vi "Actor Core.vi"(8 "error in":errorcluster, 11 "Nested in":refnum<class "UI_Up_Down.lvclass">) -> (0 "error out":errorcluster, 3 "Actor out":refnum<class "Actor.lvclass">)   [LabVIEW 2021, in "UI_Up_Down.lvclass"]
doc: "(<B>Filename</B>: Actor Framework.lvlib:Actor.lvclass:Actor Core.vi)\n\nReceives messages to the actor, reacts to them, and initiates any error handling that may shut the actor down.\n\nDescendant classes may override this VI to append parallel tasks for the actor to complete while it handles messages. Overrides use the Call Parent Method node."
uses:
  UI_Up_Down.lvclass
  C:/Program Files (x86)/National Instruments/LabVIEW 2021/user.lib/John_Lib/AbstractActorTemplate/AbstractActorTemplate/UIActorTop.lvclass
  C:/Program Files (x86)/National Instruments/LabVIEW 2021/vi.lib/ActorFramework/Actor/Actor.lvclass
  <vilib>/ActorFramework/Actor/Actor.lvclass
  UI_Up_Down.lvclass/UI_Up_Down.ctl
  <vilib>/ActorFramework/Actor/Actor.lvclass/Actor.ctl
  <vilib>/ActorFramework/Message Enqueuer/Message Enqueuer.lvclass/Message Enqueuer.ctl
  <vilib>/ActorFramework/Message Enqueuer/Init from Existing Queue.vi
  <vilib>/ActorFramework/Message Enqueuer/Enqueue.vi
  <vilib>/ActorFramework/Stop Msg/Stop Msg.lvclass
  C:/Program Files (x86)/National Instruments/LabVIEW 2021/vi.lib/ActorFramework/Message/Message.lvclass
  <vilib>/Utility/LVClass/Get LV Class Name.vi
  <resource>/AFDebug/Generate Trace for Message.vi
  <vilib>/ActorFramework/Message Priority Queue/Priority Enqueue.vi
  <vilib>/ActorFramework/Message Enqueuer/Message Enqueuer.lvclass
  <userlib>/John_Lib/AbstractActorTemplate/AbstractActorTemplate/UIActorTop.lvclass
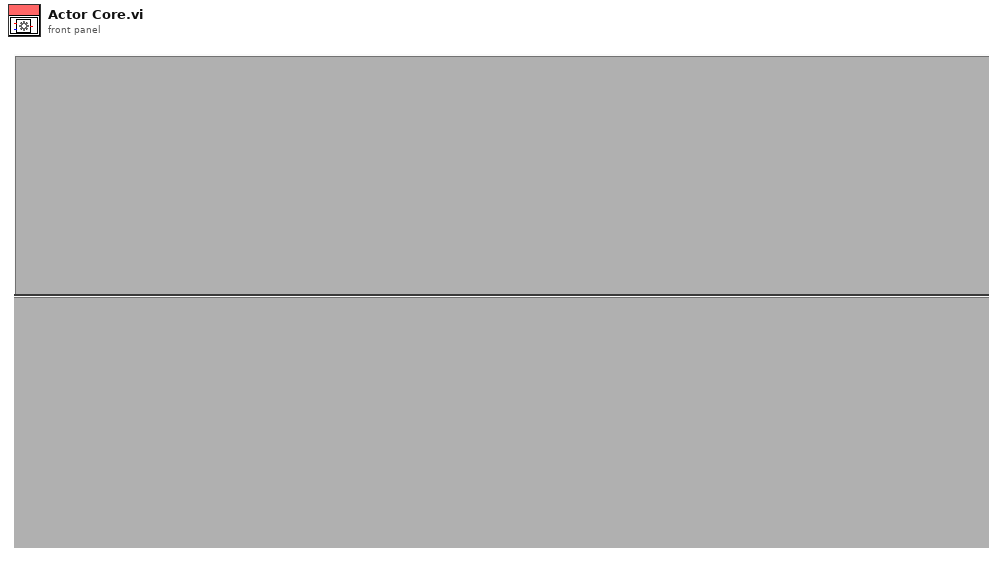
[diagram p1: front panel]
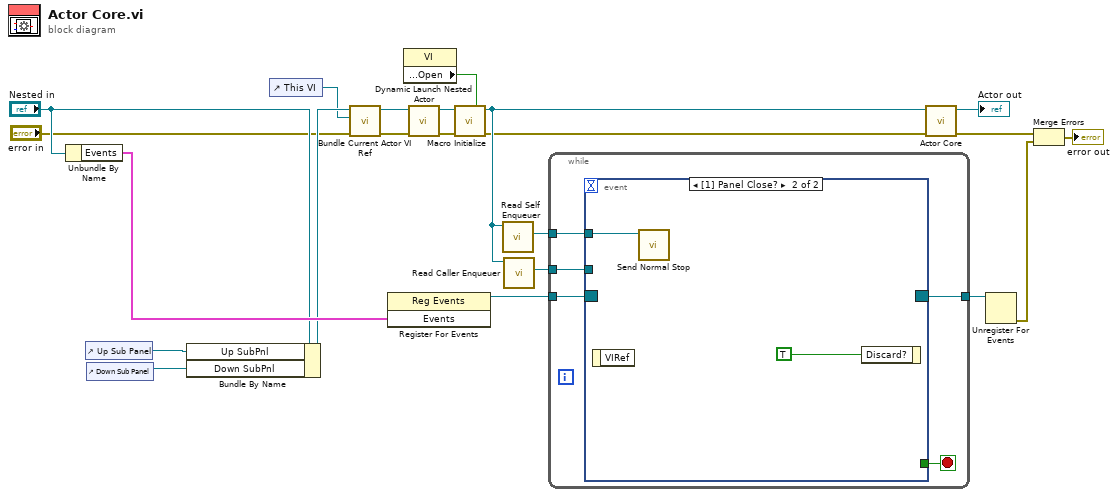
[diagram p0: block diagram]
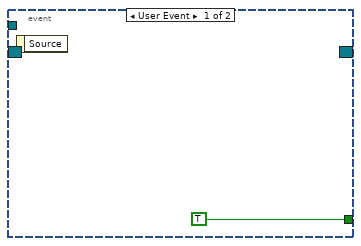
[diagram p2: hidden frame]
diagram:
  n1 = Unbundle By Name("Nested in") -> ("Events"=w20:cluster{"Stop":refnum<user-event>})
  n2 = control-ref of="Up Sub Panel"() -> (w6:refnum<vi>)
  n3 = control-ref of="Down Sub Panel"() -> (w5:refnum<vi>)
  n4 = Bundle By Name(cluster="Nested in", "Up SubPnl"=w6, "Down SubPnl"=w5) -> (w7:refnum<class "UI_Up_Down.lvclass">)
  n5 = control-ref of="This VI"() -> (w2:refnum<vi>)
  n6 = call <userlib>:"Bundle Current Actor VI Ref.vi"("error in (no error)"="error in", "This VI"=w2, "UI ActorTop in"=w7) -> ("error out"=w8:errorcluster, "UI ActorTop out"=w9:refnum<class "UI_Up_Down.lvclass">)  [unwired: 5 in, 2 out]
  n7 = register-events ("Main Register for Events")(w20) -> (reference out=w21:refnum<event-registration>)  [unwired: 2 in, 1 out]
  n8 = property class="VI"() -> ("Front Panel.Open"=w16:bool)  [unwired: 2 in, 2 out]
  n9 = call-dynamic "Dynamic Launch Nested Actor.vi"("error in (no error)"=w8, "UI ActorTop in"=w9) -> ("error out"=w17:errorcluster, "UI ActorTop out"=w18:refnum<class "UI_Up_Down.lvclass">)  [unwired: 8 in]
  n10 = call-dynamic "Macro Initialize.vi"("Front Panel Window:Open"=w16, "error in (no error)"=w17, "UI ActorTop in"=w18) -> ("error out"=w11:errorcluster, "UI ActorTop out"=w15:refnum<class "UI_Up_Down.lvclass">)  [unwired: 7 in]
  n11 = call <vilib>:"Read Self Enqueuer.vi"("Actor"=w15) -> ("Self Enqueuer"=w4:refnum<class "Message Enqueuer.lvclass">)  [unwired: 10 in]
  n12 = call <vilib>:"Read Caller Enqueuer.vi"("Actor"=w15) -> ("Caller Enqueuer"=w3:refnum<class "Message Enqueuer.lvclass">)  [unwired: 10 in]
  n13 = while {
    tunnel: w21 -> [w27]
    tunnel: [w25] -> w19
    tunnel: w4 -> [w24]
    tunnel: w3 -> [w23]
    stop <- w26 stop-if-true
    n14 = event "UI Events" shown="[1] Panel Close?" {
      selector: w27 -> [_ _]
      dyn-events: [_ _] -> w25
      timeout: _ -> [_ _]
      tunnel: [TRUE _] -> w26
      tunnel: w24 -> [_ w29]
      tunnel: w23 -> [_ _]
      event User Event {
        n15 = event-data() -> ()  [unwired: 1 in, 1 out]
      }
      event Panel Close? {
        n16 = event-data() -> ()  [unwired: 1 in, 1 out]
        n17 = call <vilib>:"Send Normal Stop.vi"("Message Enqueuer"=w29) -> ()  [unwired: 10 in, 1 out]
        n18 = event-data("Discard?"=TRUE) -> ()  [unwired: 1 in, 1 out]
      }
    }
  }
  n19 = call-parent "Actor Core.vi"("error in"=w11, "Actor in"=w15) -> ("error out"=w13:errorcluster, "Actor out"=→"Actor out":refnum<class "Actor.lvclass">)  [unwired: 8 in]
  n20 = Unregister For Events(event registration refnum=w19) -> (error out=w14:errorcluster)  [unwired: 1 in]
  n21 = Merge Errors(w13, w14) -> (→"error out":errorcluster)
